vi "DC_offset.vi"(8 "Duration":dbl, 9 "Ampltude":dbl, 10 "Position":dbl format="%#_13g", 11 "Sine":sgl[](array[numeric])) -> (3 "Sine+Anomaly":sgl[](graph))   [LabVIEW 2020]
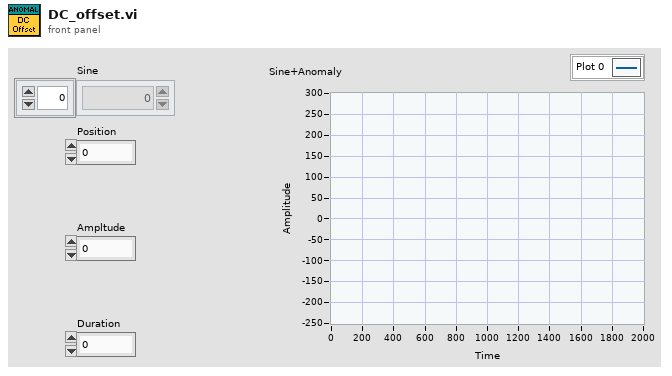
[diagram p1: front panel]
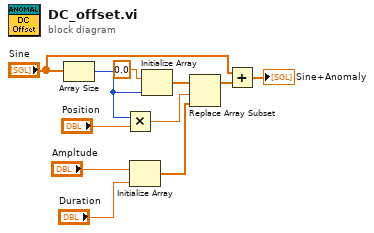
[diagram p0: block diagram]
diagram:
  n1 = Array Size(array="Sine") -> (size(s)=w6:i32)
  n2 = Multiply(x=w6, y="Position") -> (x*y=w1:dbl)
  n3 = Initialize Array("Ampltude", "Duration") -> (w9:dbl[])
  n4 = Initialize Array(sgl 0.0 ("element"), w6) -> (w8:sgl[])
  n5 = Replace Array Subset(array=w8, new element=w9, index=w1) -> (w10:sgl[])
  n6 = Add(x="Sine", y=w10) -> (x+y=→"Sine+Anomaly":sgl[])
